vi "GetFileCreationDate.vi"(9 "File Path":path) -> (0 "Error":bool, 3 "File Created Date (UTC)":timestamp)   [LabVIEW 2022 SP3]
uses:
  kernel32.dll
panel:
  in  "date time rec":T1
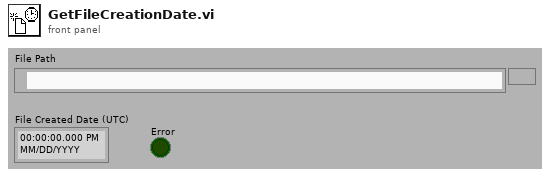
[diagram p1: front panel]
types:
  T1 = cluster{"fractional second":dbl, "second":i32, "minute":i32, "hour":i32, "day of month":i32, "month":i32, "year":i32, "day of week":i32, "day of year":i32, "DST":i32}
  T2 = cluster{"wYear":u16, "wMonth":u16, "wDayOfWeek":u16, "wDay":u16, "wHour":u16, "wMinute":u16, "wSeconds":u16, "wMilliseconds":u16}
  T3 = cluster{"dwFileAttributes":i32, "ftCreationTime":cluster{"dwLowDateTime":i32, "dwHighDateTime":i32}, "ftLastAccessTime":cluster{"dwLowDateTime":i32, "dwHighDateTime":i32}, "ftLastWrittenTime":cluster{"dwLowDateTime":i32, "dwHighDateTime":i32}, "nFileSizeHigh":i32, "nFileSizeLow":i32}
  T4 = cluster{"dwLowDateTime":i32, "dwHighDateTime":i32}
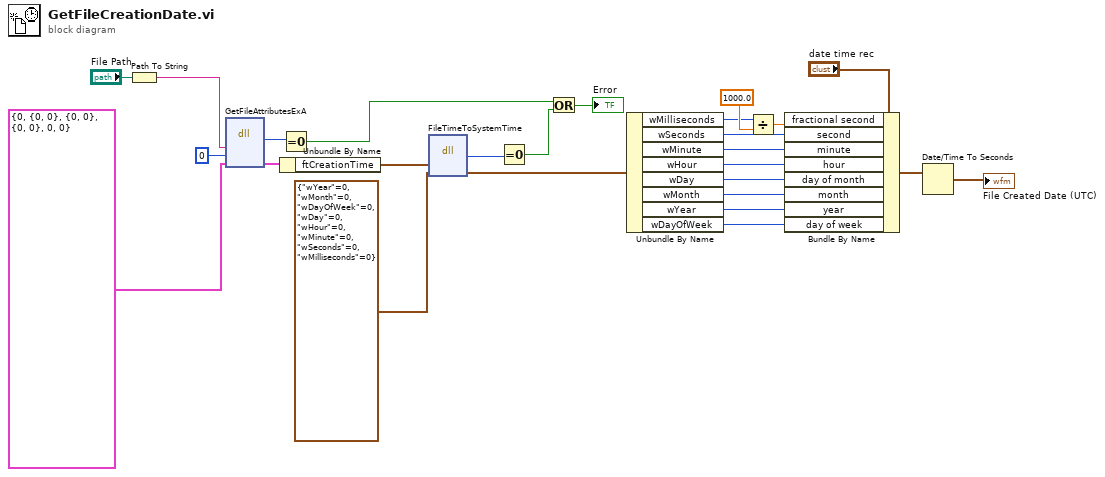
[diagram p0: block diagram]
diagram:
  n1 = Path To String(path="File Path") -> (string=w25:string)
  n2 = dll-call lib="kernel32.dll" fn="GetFileAttributesExA" label="GetFileAttributesEx"("lpFileName"=w25, "fInfoLevelID"=0, "output param"=T3 {"dwFileAttributes"=0, "ftCreationTime"={"dwLowDateTime"=0, "dwHighDateTime"=0}, "ftLastAccessTime"={"dwLowDateTime"=0, "dwHighDateTime"=0}, "ftLastWrittenTime"={"dwLowDateTime"=0, "dwHighDateTime"=0}, "nFileSizeHigh"=0, "nFileSizeLow"=0}) -> (w19:i32, "output param"=w22:T3)  [unwired: 5 in, 2 out]
  n3 = Unbundle By Name(w22) -> ("ftCreationTime"=w21:T4)
  n4 = Equal To 0?(x=w19) -> (x = 0?=w16:bool)
  n5 = dll-call lib="kernel32.dll" fn="FileTimeToSystemTime"("ftCreationTime"=w21, "output param"=T2 {"wYear"=0, "wMonth"=0, "wDayOfWeek"=0, "wDay"=0, "wHour"=0, "wMinute"=0, "wSeconds"=0, "wMilliseconds"=0}) -> (w18:i32, "output param"=w14:T2)  [unwired: 4 in, 2 out]
  n6 = Equal To 0?(x=w18) -> (x = 0?=w17:bool)
  n7 = Or(x=w16, y=w17) -> (x .or. y?=→"Error":bool)
  n8 = Unbundle By Name(w14) -> ("wMilliseconds"=w3:u16, "wSeconds"=w13:u16, "wMinute"=w12:u16, "wHour"=w11:u16, "wDay"=w10:u16, "wMonth"=w9:u16, "wYear"=w8:u16, "wDayOfWeek"=w7:u16)
  n9 = Divide(x=w3, y=1000.0) -> (x/y=w2:dbl)
  n10 = Bundle By Name(cluster="date time rec", "fractional second"=w2, "second"=w13, "minute"=w12, "hour"=w11, "day of month"=w10, "month"=w9, "year"=w8, "day of week"=w7) -> (w1:T1)
  n11 = Date/Time To Seconds(2:w1) -> (0:→"File Created Date (UTC)":timestamp)  [unwired: 1 in]
